vi "GetCalculateScanningParameter.vi"() -> ()   [LabVIEW 2011]
panel:
  in  "AmplitudeFactor":dbl
  in  "WaveTableRate":dbl
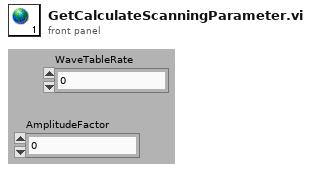
[diagram p1: front panel]
diagram:
